vi "Select List Items.vi"(4 "Item Names":string[](array[string])) -> (1 "Selected Items":string[](array[string]))   [LabVIEW 2022 SP3]
panel:
  in  "OK Button":bool
  in  "Listbox":i32[](listbox)
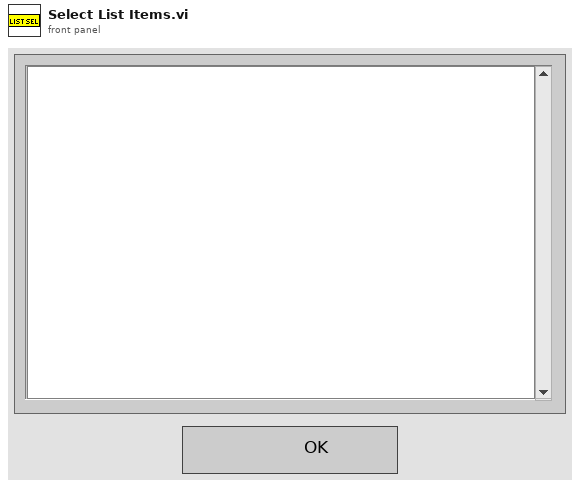
[diagram p1: front panel]
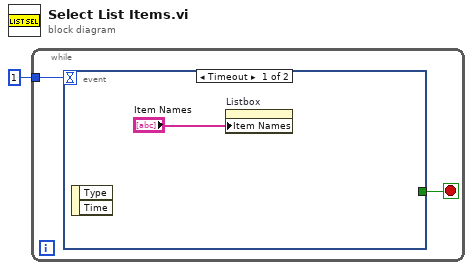
[diagram p0: block diagram]
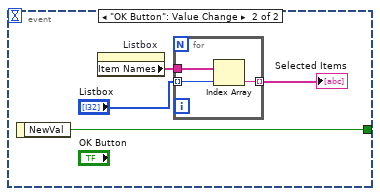
[diagram p2: hidden frame]
diagram:
  n1 = while {
    tunnel: 1 -> [w3]
    stop <- w2 stop-if-true
    n2 = event shown="[0] Timeout" {
      selector: _ -> [_ _]
      dyn-events: _ -> [_ _]
      timeout: w3 -> [_ _]
      tunnel: [_ w8] -> w2
      event Timeout {
        n3 = event-data() -> ()  [unwired: 1 in, 2 out]
        n4 = property on="Listbox" class="LstBox (strict)"("Item Names"="Item Names") -> ()  [unwired: 2 in, 2 out]
      }
      event "OK Button": Value Change {
        n5 = event-data() -> ("NewVal"=w8:bool)  [unwired: 1 in]
        n6 = property on="Listbox" class="LstBox (strict)"() -> ("Item Names"=w6:string[])  [unwired: 2 in, 2 out]
        n7 = for {
          tunnel: "Listbox" -> [w11] mode=indexing
          tunnel: w6 -> [w10]
          tunnel: [w9] -> w5 mode=indexing
          n8 = Index Array(array=w10, index=w11) -> (element=w9:string)
        }
        "Selected Items" <- w5
      }
    }
  }
